vi "Change Setting.vi"(8 "error in (no error)":errorcluster, 10 "Change setting mode":T1=enum."Next", 11 "Toggle 8 in":refnum<class "Toggle 8.lvclass">) -> (0 "error out":errorcluster, 1 "Changes":cluster{"Name":string, "Value":string}[](array[cluster]), 2 "Last setting":bool, 3 "Toggle 8 out":refnum<class "Toggle 8.lvclass">)   [LabVIEW 2020, in "Toggle 8.lvclass"]
uses:
  Toggle 8.lvclass
  Controls/Change setting mode enum.ctl
  Controls/Register to Write.ctl
  PIC-device/PIC-Device.lvclass
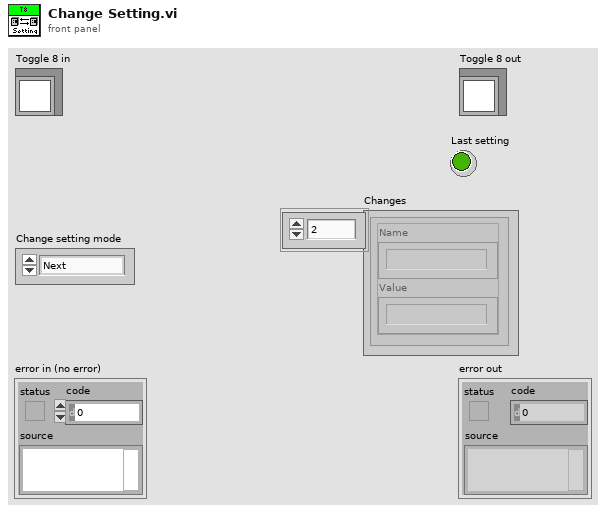
[diagram p1: front panel]
types:
  T1 = typedef "PIC-Device.lvclass/Change setting mode enum.ctl" = enum16{"Init", "Next", "Reset"}
  T2 = typedef "Toggle 8.lvclass/Test Sequence.ctl" = cluster{"CP values":string, "Charge Pump values":enum16{"CP 24V", "CP 26V", "CP 28V", "CP 30V", "CP 31V", "CP 32V", "CP 33V", "CP 34V", "CP 35V", "CP 36V", "CP 37V", "CP 38V", "CP 39V", "CP 40V", "CP 41V", "CP 42V", "CP 43V", "CP 44V", "CP 45V", "CP 46V", "CP 47V", "CP 48V", "CP 49V", "CP 50V", "CP 51V", "CP 52V", "CP 53V", "CP 54V", "CP 56V", "CP 58V", "CP 60V", "CP 62V"}[], "Charge Pump":T3[], "Control individual beams":bool, "OTP/beam values":dbl[], "Capa settings":T3[], "OTP Values string":string}
  T3 = typedef "PIC-Device.lvclass/Register to Write.ctl" = cluster{"Register":u32, "Value":u32, "Dev Address":u32, "Physical Adress":u32}
  T4 = enum16{"CP 24V", "CP 26V", "CP 28V", "CP 30V", "CP 31V", "CP 32V", "CP 33V", "CP 34V", "CP 35V", "CP 36V", "CP 37V", "CP 38V", "CP 39V", "CP 40V", "CP 41V", "CP 42V", "CP 43V", "CP 44V", "CP 45V", "CP 46V", "CP 47V", "CP 48V", "CP 49V", "CP 50V", "CP 51V", "CP 52V", "CP 53V", "CP 54V", "CP 56V", "CP 58V", "CP 60V", "CP 62V"}[]
  T5 = enum16{"CP 24V", "CP 26V", "CP 28V", "CP 30V", "CP 31V", "CP 32V", "CP 33V", "CP 34V", "CP 35V", "CP 36V", "CP 37V", "CP 38V", "CP 39V", "CP 40V", "CP 41V", "CP 42V", "CP 43V", "CP 44V", "CP 45V", "CP 46V", "CP 47V", "CP 48V", "CP 49V", "CP 50V", "CP 51V", "CP 52V", "CP 53V", "CP 54V", "CP 56V", "CP 58V", "CP 60V", "CP 62V"}
  T6 = cluster{"Register":bool, "Value":bool, "Dev Address":bool, "Physical Adress":bool}
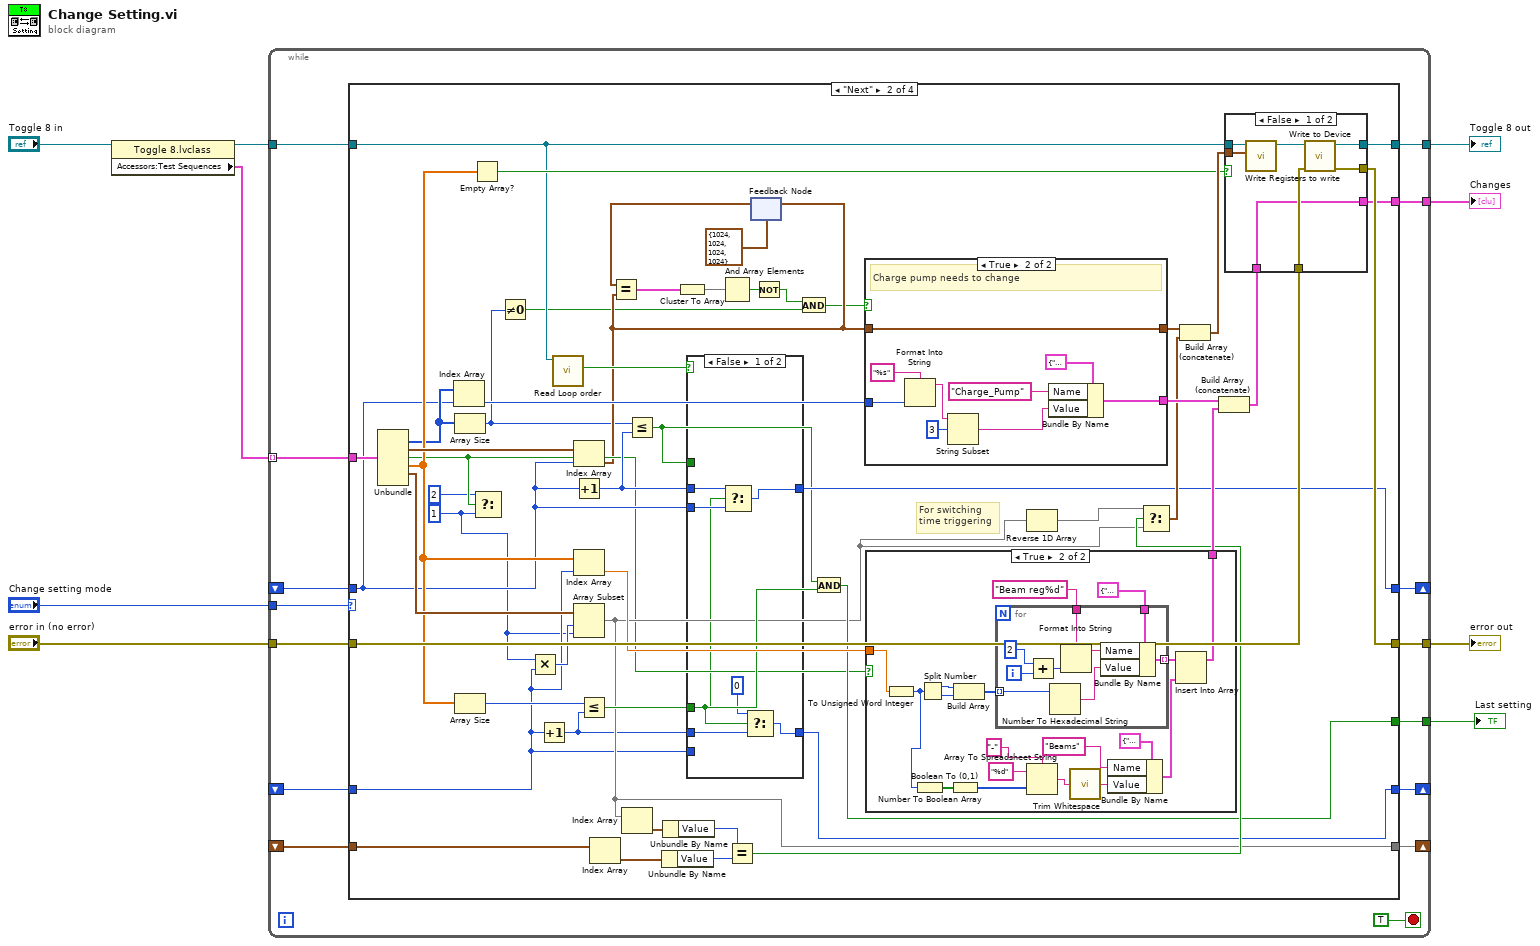
[diagram p0: block diagram]
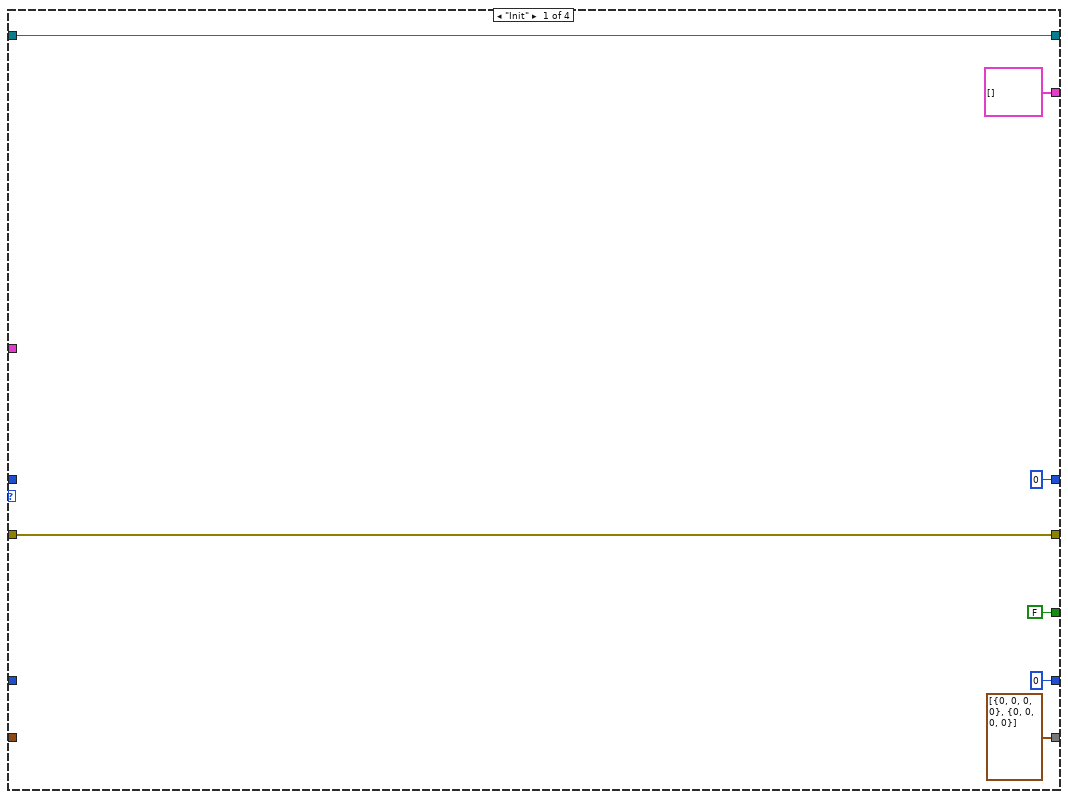
[diagram p2: hidden frame]
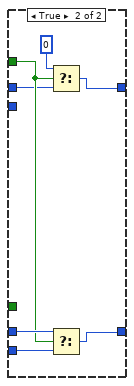
[diagram p3: hidden frame]
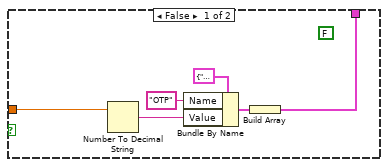
[diagram p4: hidden frame]
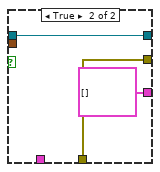
[diagram p6: hidden frame]
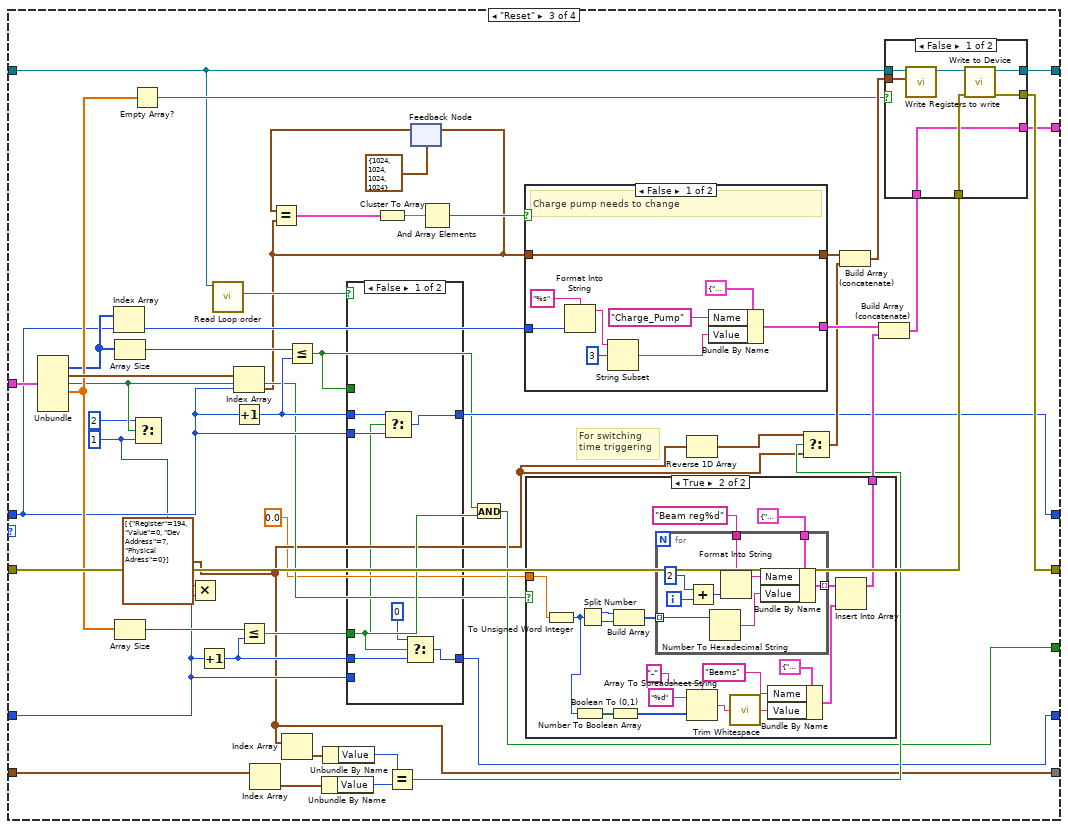
[diagram p7: hidden frame]
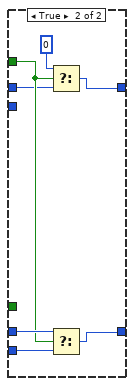
[diagram p8: hidden frame]
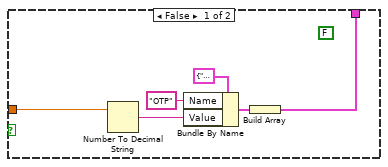
[diagram p9: hidden frame]
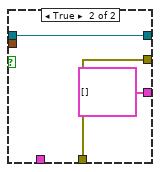
[diagram p11: hidden frame]
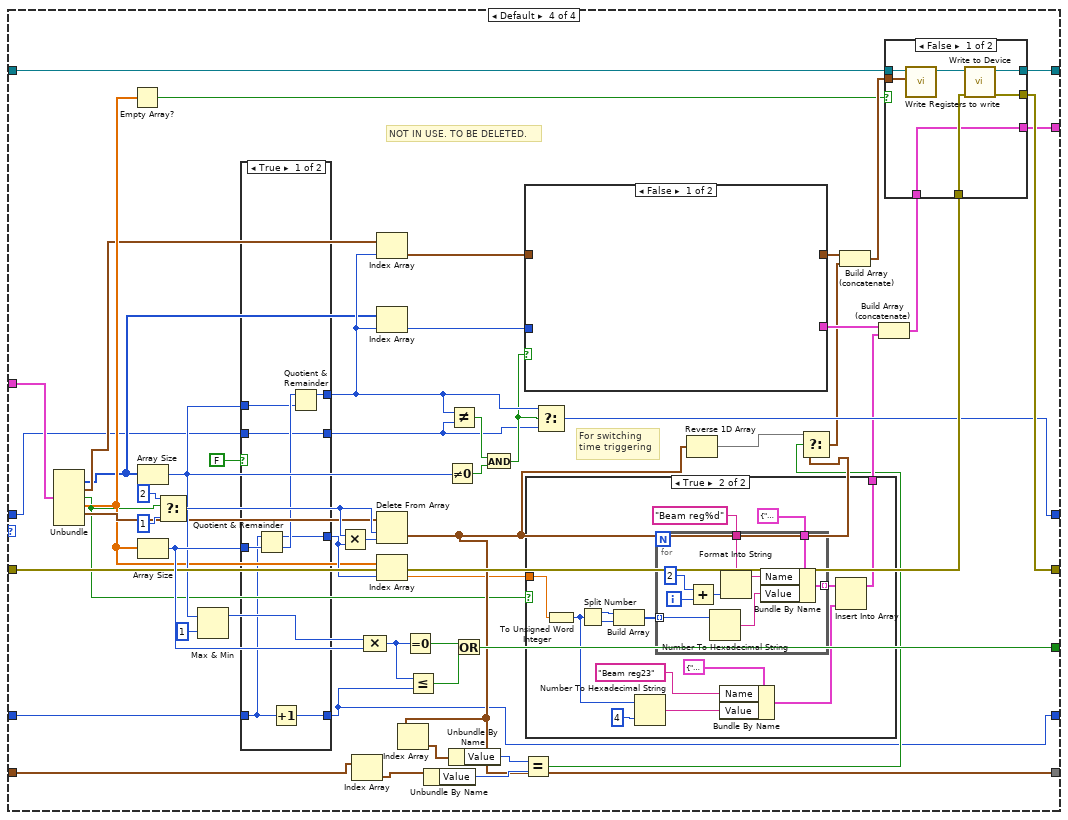
[diagram p12: hidden frame]
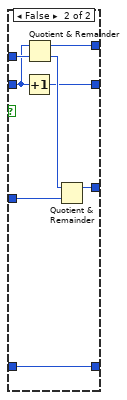
[diagram p13: hidden frame]
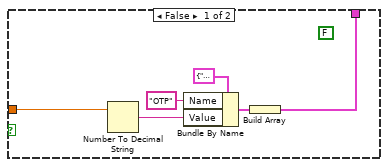
[diagram p14: hidden frame]
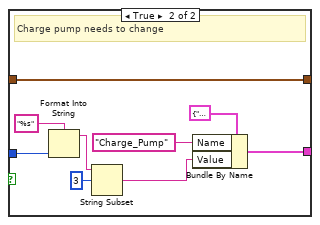
[diagram p15: hidden frame]
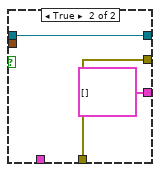
[diagram p16: hidden frame]
diagram:
  n1 = property class="Toggle 8.lvclass"(reference="Toggle 8 in") -> (reference out=w6:refnum<class "Toggle 8.lvclass">, "Accessors:Test Sequences"=w8:T2[])  [unwired: 1 in, 1 out]
  n2 = while {
    tunnel: w8 -> [w24] mode=indexing
    tunnel: "Change setting mode" -> [w22]
    shift-right: [w10] -> _
    shift-left: _ -> [w11]
    shift-right: [w21] -> _
    shift-left: _ -> [w20]
    tunnel: w6 -> [w19]
    tunnel: [w18] -> w5
    tunnel: [w17] -> w4
    tunnel: "error in (no error)" -> [w16]
    tunnel: [w15] -> w2
    tunnel: [w14] -> w1
    shift-right: [w13] -> _
    shift-left: _ -> [w12]
    stop <- TRUE stop-if-true
    n3 = case shown="\"Next\"" w22 {
      tunnel: w24 -> [_ w83 w196 w314]
      tunnel: [0 w49 w165 w264] -> w10
      tunnel: w11 -> [_ w46 w162 w265]
      tunnel: [0 w56 w170 w305] -> w21
      tunnel: w20 -> [_ w57 w171 w266]
      tunnel: w19 -> [w26 w45 w161 w311]
      tunnel: [w26 w80 w193 w310] -> w18
      tunnel: [FALSE w60 w174 w296] -> w17
      tunnel: w16 -> [w28 w79 w192 w308]
      tunnel: [w28 w78 w191 w307] -> w15
      tunnel: [cluster{"Name":string, "Value":string}[] [] w75 w188 w300] -> w14
      tunnel: [T3[] [{"Register"=0, "Value"=0, "Dev Address"=0, "Physical Adress"=0}, {"Register"=0, "Value"=0, "Dev Address"=0, "Physical Adress"=0}] ("Capa settings") w55 w151 w275] -> w13
      tunnel: w12 -> [_ w71 w184 w280]
      frame "Init" {
      }
      frame "Next" {
        w37 = 1
        # "For switching \ntime triggering"
        n4 = Unbundle(w83) -> ("Charge Pump values"=w62:T4, "Charge Pump"=w64:T3[], "Control individual beams"=w53:bool, "OTP/beam values"=w63:dbl[], "Capa settings"=w65:T3[])  [unwired: 2 out]
        n5 = Index Array(array=w62, index=w57) -> (element=w50:T5)
        n6 = Array Size(array=w62) -> (size(s)=w36:i32)
        n7 = Array Size(array=w63) -> (size(s)=w61:i32)
        n8 = Empty Array?(array=w63) -> (empty?=w81:bool)
        n9 = Select(t=2, s=w53, f=w37) -> ()  [unwired: 1 out]
        n10 = Not Equal To 0?(x=w36) -> (x != 0?=w35:bool)
        n11 = Multiply(x=w37, y=w46) -> (x*y=w51:i32)
        n12 = Increment(x=w46) -> (x+1=w48:i32)
        n13 = call-dynamic "Read Loop order.vi"("Toggle 8 in"=w45) -> ("Loop order"=w44:bool)  [unwired: 9 in, 1 out]
        n14 = Index Array(array=w64, index=w57) -> (element=w38:T3)
        n15 = Increment(x=w57) -> (x+1=w58:i32)
        n16 = Index Array(array=w63, index=w46) -> (element=w66:dbl)
        n17 = Array Subset(array=w65, index=w51, length=w37) -> (w55:T3[])
        n18 = Less Or Equal?(x=w61, y=w48) -> (x <= y?=w59:bool)
        n19 = Index Array(array=w71) -> (element=w70:T3)  [unwired: 1 in]
        n20 = Index Array(array=w55) -> (element=w54:T3)  [unwired: 1 in]
        n21 = Less Or Equal?(x=w36, y=w58) -> (x <= y?=w47:bool)
        n22 = Unbundle By Name(w70) -> ("Value"=w69:u32)
        n23 = Unbundle By Name(w54) -> ("Value"=w68:u32)
        n24 = case shown="False" w44 {
          tunnel: w59 -> [w87 _]
          tunnel: w58 -> [w90 w93]
          tunnel: w57 -> [w89 _]
          tunnel: [w84 w92] -> w56
          tunnel: [w85 w95] -> w49
          tunnel: w48 -> [w86 w97]
          tunnel: w46 -> [_ w96]
          tunnel: w47 -> [_ w94]
          frame False {
            n25 = Select(t=w90, s=w87, f=w89) -> (s? t:f=w84:i32)
            n26 = Select(t=0, s=w87, f=w86) -> (s? t:f=w85:i32)
          }
          frame True {
            n27 = Select(t=0, s=w94, f=w93) -> (s? t:f=w92:i32)
            n28 = Select(t=w97, s=w94, f=w96) -> (s? t:f=w95:i32)
          }
        }
        n29 = Equal?(x=w68, y=w69) -> (x = y?=w67:bool)
        n30 = feedback-in #1(w38) -> ()
        n31 = feedback #1(T3 {"Register"=1024, "Value"=1024, "Dev Address"=1024, "Physical Adress"=1024} ("reg cluster")) -> (w42:T3)
        n32 = Equal?(x=w42, y=w38) -> (x = y?=w41:T6)
        n33 = Cluster To Array(cluster=w41) -> (array=w40:bool[])
        n34 = And Array Elements(Boolean array=w40) -> (logical AND=w33:bool)
        n35 = Not(x=w33) -> (.not. x?=w32:bool)
        n36 = And(x=w32, y=w35) -> (x .and. y?=w34:bool)
        n37 = And(x=w47, y=w59) -> (x .and. y?=w60:bool)
        n38 = case shown="True" w34 {
          tunnel: w38 -> [_ w137]
          tunnel: w50 -> [_ w134]
          tunnel: [_ w137] -> w43
          tunnel: [_ w136] -> w77
          frame False {
          }
          frame True {
            # "Charge pump needs to change"
            n39 = Format Into String(format string="%s", w134) -> (resulting string=w133:string)  [unwired: 2 in, 1 out]
            n40 = String Subset(string=w133, offset (0)=3) -> (substring=w131:string)  [unwired: 1 in]
            n41 = Bundle By Name(cluster=cluster{"Name":string, "Value":string} {"Name"="", "Value"=""} ("Change"), "Name"="Charge_Pump", "Value"=w131) -> (w136:cluster{"Name":string, "Value":string})
          }
        }
        n42 = case shown="True" w53 {
          tunnel: [w101 w111] -> w74
          tunnel: w66 -> [w98 w117]
          frame False {
            (unwired) FALSE
            n43 = Number To Decimal String(number=w98) -> (decimal integer string=w99:string)  [unwired: 1 in]
            n44 = Bundle By Name(cluster=cluster{"Name":string, "Value":string} {"Name"="", "Value"=""} ("Change"), "Name"="OTP", "Value"=w99) -> (w102:cluster{"Name":string, "Value":string})
            n45 = Build Array(w102) -> (w101:cluster{"Name":string, "Value":string}[])
          }
          frame True {
            n46 = To Unsigned Word Integer(number=w117) -> (unsigned 16bit integer=w106:u16)
            n47 = Number To Boolean Array(number=w106) -> (Boolean array=w109:bool[])
            n48 = Split Number(x=w106) -> (hi(x)=w118:u8, lo(x)=w119:u8)
            n49 = Boolean To (0,1)(Boolean=w109) -> (0, 1=w110:i16[])
            n50 = Build Array(w118, w119) -> (w116:u8[])
            n51 = for {
              tunnel: cluster{"Name":string, "Value":string} {"Name"="", "Value"=""} ("Change") -> [w130]
              tunnel: [w129] -> w112 mode=indexing
              tunnel: "Beam reg%d" ("Name") -> [w128]
              tunnel: w116 -> [w122] mode=indexing
              i -> [w127]
              n52 = Add(x=2, y=w127) -> (x+y=w125:i32)
              n53 = Number To Hexadecimal String(2:w122) -> (0:w123:string)  [unwired: 1 in]
              n54 = Format Into String(format string=w128, w125) -> (resulting string=w124:string)  [unwired: 2 in, 1 out]
              n55 = Bundle By Name(cluster=w130, "Name"=w124, "Value"=w123) -> (w129:cluster{"Name":string, "Value":string})
            }
            n56 = Array To Spreadsheet String(delimiter (Tab)="-", array=w110, 3:"%d" ("format string")) -> (spreadsheet string=w105:string)
            n57 = call <vilib>:"Trim Whitespace.vi"("string"=w105) -> ("trimmed string"=w104:string)  [unwired: 1 in]
            n58 = Bundle By Name(cluster=cluster{"Name":string, "Value":string} {"Name"="", "Value"=""} ("Change"), "Name"="Beams", "Value"=w104) -> (w113:cluster{"Name":string, "Value":string})
            n59 = Insert Into Array(array=w112, new element=w113) -> (w111:cluster{"Name":string, "Value":string}[])  [unwired: 1 in]
          }
        }
        n60 = Reverse 1D Array(array=w55) -> (reversed array=w73:T3[])
        n61 = Select(t=w73, s=w67, f=w55) -> (s? t:f=w72:T3[])
        n62 = Build Array (concatenate)(w43, w72) -> (w82:T3[])
        n63 = Build Array (concatenate)(w77, w74) -> (w76:cluster{"Name":string, "Value":string}[])
        n64 = case shown="False" w81 {
          tunnel: w45 -> [w146 w149]
          tunnel: w82 -> [w145 _]
          tunnel: [w143 w149] -> w80
          tunnel: [w142 w147] -> w78
          tunnel: [w140 cluster{"Name":string, "Value":string}[] []] -> w75
          tunnel: w79 -> [w141 w147]
          tunnel: w76 -> [w140 _]
          frame False {
            n65 = call-dynamic "Write Registers to write.vi"("Registers to write"=w145, "Device in"=w146) -> ("Device out"=w144:refnum<class "Toggle 8.lvclass">)  [unwired: 9 in]
            n66 = call-dynamic "Write to Device.vi"("error in (no error)"=w141, "Device in"=w144) -> ("error out"=w142:errorcluster, "Device out"=w143:refnum<class "Toggle 8.lvclass">)  [unwired: 7 in, 1 out]
          }
          frame True {
          }
        }
      }
      frame "Reset" {
        w151 = T3[] [{"Register"=194, "Value"=0, "Dev Address"=7, "Physical Adress"=0}] ("Capa settings")
        w152 = 1
        # "For switching \ntime triggering"
        n67 = Unbundle(w196) -> ("Charge Pump values"=w177:T4, "Charge Pump"=w179:T3[], "Control individual beams"=w168:bool, "OTP/beam values"=w178:dbl[])  [unwired: 3 out]
        n68 = Index Array(array=w177, index=w171) -> (element=w166:T5)
        n69 = Array Size(array=w177) -> (size(s)=w175:i32)
        n70 = Array Size(array=w178) -> (size(s)=w176:i32)
        n71 = Empty Array?(array=w178) -> (empty?=w194:bool)
        n72 = Select(t=2, s=w168, f=w152) -> ()  [unwired: 1 out]
        n73 = Multiply(x=w152, y=w162) -> ()  [unwired: 1 out]
        n74 = Increment(x=w162) -> (x+1=w164:i32)
        n75 = call-dynamic "Read Loop order.vi"("Toggle 8 in"=w161) -> ("Loop order"=w160:bool)  [unwired: 9 in, 1 out]
        n76 = Index Array(array=w179, index=w171) -> (element=w153:T3)
        n77 = Increment(x=w171) -> (x+1=w172:i32)
        n78 = Less Or Equal?(x=w176, y=w164) -> (x <= y?=w173:bool)
        n79 = Index Array(array=w184) -> (element=w183:T3)  [unwired: 1 in]
        n80 = Index Array(array=w151) -> (element=w169:T3)  [unwired: 1 in]
        n81 = Less Or Equal?(x=w175, y=w172) -> (x <= y?=w163:bool)
        n82 = Unbundle By Name(w183) -> ("Value"=w182:u32)
        n83 = Unbundle By Name(w169) -> ("Value"=w181:u32)
        n84 = case shown="False" w160 {
          tunnel: w173 -> [w200 _]
          tunnel: w172 -> [w203 w206]
          tunnel: w171 -> [w202 _]
          tunnel: [w197 w205] -> w170
          tunnel: [w198 w208] -> w165
          tunnel: w164 -> [w199 w210]
          tunnel: w162 -> [_ w209]
          tunnel: w163 -> [_ w207]
          frame False {
            n85 = Select(t=w203, s=w200, f=w202) -> (s? t:f=w197:i32)
            n86 = Select(t=0, s=w200, f=w199) -> (s? t:f=w198:i32)
          }
          frame True {
            n87 = Select(t=0, s=w207, f=w206) -> (s? t:f=w205:i32)
            n88 = Select(t=w210, s=w207, f=w209) -> (s? t:f=w208:i32)
          }
        }
        n89 = Equal?(x=w181, y=w182) -> (x = y?=w180:bool)
        n90 = feedback-in #2(w153) -> ()
        n91 = feedback #2(T3 {"Register"=1024, "Value"=1024, "Dev Address"=1024, "Physical Adress"=1024} ("reg cluster")) -> (w158:T3)
        n92 = Equal?(x=w158, y=w153) -> (x = y?=w157:T6)
        n93 = Cluster To Array(cluster=w157) -> (array=w156:bool[])
        n94 = And Array Elements(Boolean array=w156) -> (logical AND=w155:bool)
        n95 = And(x=w163, y=w173) -> (x .and. y?=w174:bool)
        n96 = case shown="False" w155 {
          tunnel: w153 -> [w250 _]
          tunnel: w166 -> [w247 _]
          tunnel: [w250 _] -> w159
          tunnel: [w249 _] -> w190
          frame False {
            # "Charge pump needs to change"
            n97 = Format Into String(format string="%s", w247) -> (resulting string=w246:string)  [unwired: 2 in, 1 out]
            n98 = String Subset(string=w246, offset (0)=3) -> (substring=w244:string)  [unwired: 1 in]
            n99 = Bundle By Name(cluster=cluster{"Name":string, "Value":string} {"Name"="", "Value"=""} ("Change"), "Name"="Charge_Pump", "Value"=w244) -> (w249:cluster{"Name":string, "Value":string})
          }
          frame True {
          }
        }
        n100 = case shown="True" w168 {
          tunnel: [w214 w224] -> w187
          tunnel: 0.0 ("OTP/beam value") -> [w211 w230]
          frame False {
            (unwired) FALSE
            n101 = Number To Decimal String(number=w211) -> (decimal integer string=w212:string)  [unwired: 1 in]
            n102 = Bundle By Name(cluster=cluster{"Name":string, "Value":string} {"Name"="", "Value"=""} ("Change"), "Name"="OTP", "Value"=w212) -> (w215:cluster{"Name":string, "Value":string})
            n103 = Build Array(w215) -> (w214:cluster{"Name":string, "Value":string}[])
          }
          frame True {
            n104 = To Unsigned Word Integer(number=w230) -> (unsigned 16bit integer=w219:u16)
            n105 = Number To Boolean Array(number=w219) -> (Boolean array=w222:bool[])
            n106 = Split Number(x=w219) -> (hi(x)=w231:u8, lo(x)=w232:u8)
            n107 = Boolean To (0,1)(Boolean=w222) -> (0, 1=w223:i16[])
            n108 = Build Array(w231, w232) -> (w229:u8[])
            n109 = for {
              tunnel: cluster{"Name":string, "Value":string} {"Name"="", "Value"=""} ("Change") -> [w243]
              tunnel: [w242] -> w225 mode=indexing
              tunnel: "Beam reg%d" ("Name") -> [w241]
              tunnel: w229 -> [w235] mode=indexing
              i -> [w240]
              n110 = Add(x=2, y=w240) -> (x+y=w238:i32)
              n111 = Number To Hexadecimal String(2:w235) -> (0:w236:string)  [unwired: 1 in]
              n112 = Format Into String(format string=w241, w238) -> (resulting string=w237:string)  [unwired: 2 in, 1 out]
              n113 = Bundle By Name(cluster=w243, "Name"=w237, "Value"=w236) -> (w242:cluster{"Name":string, "Value":string})
            }
            n114 = Array To Spreadsheet String(delimiter (Tab)="-", array=w223, 3:"%d" ("format string")) -> (spreadsheet string=w218:string)
            n115 = call <vilib>:"Trim Whitespace.vi"("string"=w218) -> ("trimmed string"=w217:string)  [unwired: 1 in]
            n116 = Bundle By Name(cluster=cluster{"Name":string, "Value":string} {"Name"="", "Value"=""} ("Change"), "Name"="Beams", "Value"=w217) -> (w226:cluster{"Name":string, "Value":string})
            n117 = Insert Into Array(array=w225, new element=w226) -> (w224:cluster{"Name":string, "Value":string}[])  [unwired: 1 in]
          }
        }
        n118 = Reverse 1D Array(array=w151) -> (reversed array=w186:T3[])
        n119 = Select(t=w186, s=w180, f=w151) -> (s? t:f=w185:T3[])
        n120 = Build Array (concatenate)(w159, w185) -> (w195:T3[])
        n121 = Build Array (concatenate)(w190, w187) -> (w189:cluster{"Name":string, "Value":string}[])
        n122 = case shown="False" w194 {
          tunnel: w161 -> [w259 w262]
          tunnel: w195 -> [w258 _]
          tunnel: [w256 w262] -> w193
          tunnel: [w255 w260] -> w191
          tunnel: [w253 cluster{"Name":string, "Value":string}[] []] -> w188
          tunnel: w192 -> [w254 w260]
          tunnel: w189 -> [w253 _]
          frame False {
            n123 = call-dynamic "Write Registers to write.vi"("Registers to write"=w258, "Device in"=w259) -> ("Device out"=w257:refnum<class "Toggle 8.lvclass">)  [unwired: 9 in]
            n124 = call-dynamic "Write to Device.vi"("error in (no error)"=w254, "Device in"=w257) -> ("error out"=w255:errorcluster, "Device out"=w256:refnum<class "Toggle 8.lvclass">)  [unwired: 7 in, 1 out]
          }
          frame True {
          }
        }
      }
      frame Default {
        # "NOT IN USE. TO BE DELETED."
        # "For switching \ntime triggering"
        n125 = Unbundle(w314) -> ("Charge Pump values"=w268:T4, "Charge Pump"=w269:T3[], "Control individual beams"=w270:bool, "OTP/beam values"=w271:dbl[], "Capa settings"=w272:T3[])  [unwired: 2 out]
        n126 = Empty Array?(array=w271) -> (empty?=w312:bool)
        n127 = Array Size(array=w268) -> (size(s)=w287:i32)
        n128 = Array Size(array=w271) -> (size(s)=w309:i32)
        n129 = Select(t=2, s=w270, f=1) -> (s? t:f=w293:i32)
        n130 = Max & Min(x=w287, y=1) -> (max(x,y)=w289:i32)  [unwired: 1 out]
        n131 = case shown="True" FALSE {
          tunnel: w309 -> [w321 w330]
          tunnel: [w320 w329] -> w292
          tunnel: [w319 w328] -> w290
          tunnel: w287 -> [w318 w327]
          tunnel: w266 -> [w316 w324]
          tunnel: w265 -> [w315 w325]
          tunnel: [w317 w325] -> w264
          tunnel: [w316 w323] -> w263
          frame True {
            n132 = Quotient & Remainder(x=w315, y=w321) -> (x-y*floor(x/y)=w320:i32, floor(x/y)=w322:i32)
            n133 = Increment(x=w315) -> (x+1=w317:i32)
            n134 = Quotient & Remainder(x=w322, y=w318) -> (x-y*floor(x/y)=w319:i32)  [unwired: 1 out]
          }
          frame False {
            n135 = Increment(x=w324) -> (x+1=w323:i32)
            n136 = Quotient & Remainder(x=w324, y=w327) -> (x-y*floor(x/y)=w328:i32, floor(x/y)=w326:i32)
            n137 = Quotient & Remainder(x=w326, y=w330) -> (x-y*floor(x/y)=w329:i32)  [unwired: 1 out]
          }
        }
        n138 = Multiply(x=w293, y=w292) -> (x*y=w291:i32)
        n139 = Index Array(array=w280) -> (element=w279:T3)  [unwired: 1 in]
        n140 = Compound Arithmetic op=MULTIPLY(w289, w309) -> (w299:i32)
        n141 = Index Array(array=w269, index=w290) -> (element=w304:T3)
        n142 = Index Array(array=w268, index=w290) -> (element=w306:T5)
        n143 = Delete From Array(array=w272, length=w293, index=w291) -> (deleted portion=w275:T3[])  [unwired: 1 out]
        n144 = Index Array(array=w271, index=w292) -> (element=w273:dbl)
        n145 = Index Array(array=w275) -> (element=w276:T3)  [unwired: 1 in]
        n146 = Equal To 0?(x=w299) -> (x = 0?=w298:bool)
        n147 = Less Or Equal?(x=w299, y=w264) -> (x <= y?=w297:bool)
        n148 = Unbundle By Name(w279) -> ("Value"=w278:u32)
        n149 = Not Equal To 0?(x=w287) -> (x != 0?=w286:bool)
        n150 = Not Equal?(x=w290, y=w263) -> (x != y?=w285:bool)
        n151 = Unbundle By Name(w276) -> ("Value"=w277:u32)
        n152 = Or(x=w298, y=w297) -> (x .or. y?=w296:bool)
        n153 = And(x=w285, y=w286) -> (x .and. y?=w284:bool)
        n154 = Equal?(x=w277, y=w278) -> (x = y?=w274:bool)
        n155 = case shown="False" w284 {
          tunnel: w304 -> [_ w366]
          tunnel: w306 -> [_ w363]
          tunnel: [_ w366] -> w303
          tunnel: [_ w365] -> w302
          frame False {
          }
          frame True {
            # "Charge pump needs to change"
            n156 = Format Into String(format string="%s", w363) -> (resulting string=w362:string)  [unwired: 2 in, 1 out]
            n157 = String Subset(string=w362, offset (0)=3) -> (substring=w360:string)  [unwired: 1 in]
            n158 = Bundle By Name(cluster=cluster{"Name":string, "Value":string} {"Name"="", "Value"=""} ("Change"), "Name"="Charge_Pump", "Value"=w360) -> (w365:cluster{"Name":string, "Value":string})
          }
        }
        n159 = case shown="True" w270 {
          tunnel: [w334 w338] -> w283
          tunnel: w273 -> [w331 w346]
          frame False {
            (unwired) FALSE
            n160 = Number To Decimal String(number=w331) -> (decimal integer string=w332:string)  [unwired: 1 in]
            n161 = Bundle By Name(cluster=cluster{"Name":string, "Value":string} {"Name"="", "Value"=""} ("Change"), "Name"="OTP", "Value"=w332) -> (w335:cluster{"Name":string, "Value":string})
            n162 = Build Array(w335) -> (w334:cluster{"Name":string, "Value":string}[])
          }
          frame True {
            n163 = To Unsigned Word Integer(number=w346) -> (unsigned 16bit integer=w337:u16)
            n164 = Split Number(x=w337) -> (hi(x)=w347:u8, lo(x)=w348:u8)
            n165 = Build Array(w347, w348) -> (w345:u8[])
            n166 = Number To Hexadecimal String(1:i16 4 ("width (-)"), 2:w337) -> (0:w343:string)
            n167 = for {
              tunnel: cluster{"Name":string, "Value":string} {"Name"="", "Value"=""} ("Change") -> [w359]
              tunnel: [w358] -> w339 mode=indexing
              tunnel: "Beam reg%d" ("Name") -> [w357]
              tunnel: w345 -> [w351] mode=indexing
              i -> [w356]
              n168 = Add(x=2, y=w356) -> (x+y=w354:i32)
              n169 = Number To Hexadecimal String(2:w351) -> (0:w352:string)  [unwired: 1 in]
              n170 = Format Into String(format string=w357, w354) -> (resulting string=w353:string)  [unwired: 2 in, 1 out]
              n171 = Bundle By Name(cluster=w359, "Name"=w353, "Value"=w352) -> (w358:cluster{"Name":string, "Value":string})
            }
            n172 = Bundle By Name(cluster=cluster{"Name":string, "Value":string} {"Name"="", "Value"=""} ("Change"), "Name"="Beam reg23", "Value"=w343) -> (w341:cluster{"Name":string, "Value":string})
            n173 = Insert Into Array(array=w339, new element=w341) -> (w338:cluster{"Name":string, "Value":string}[])  [unwired: 1 in]
          }
        }
        n174 = Select(t=w290, s=w284, f=w263) -> (s? t:f=w305:i32)
        n175 = Reverse 1D Array(array=w275) -> (reversed array=w282:T3[])
        n176 = Select(t=w282, s=w274, f=w275) -> (s? t:f=w281:T3[])
        n177 = Build Array (concatenate)(w303, w281) -> (w313:T3[])
        n178 = Build Array (concatenate)(w302, w283) -> (w301:cluster{"Name":string, "Value":string}[])
        n179 = case shown="False" w312 {
          tunnel: w311 -> [w375 w378]
          tunnel: w313 -> [w374 _]
          tunnel: [w372 w378] -> w310
          tunnel: [w371 w376] -> w307
          tunnel: [w369 cluster{"Name":string, "Value":string}[] []] -> w300
          tunnel: w308 -> [w370 w376]
          tunnel: w301 -> [w369 _]
          frame False {
            n180 = call-dynamic "Write Registers to write.vi"("Registers to write"=w374, "Device in"=w375) -> ("Device out"=w373:refnum<class "Toggle 8.lvclass">)  [unwired: 9 in]
            n181 = call-dynamic "Write to Device.vi"("error in (no error)"=w370, "Device in"=w373) -> ("error out"=w371:errorcluster, "Device out"=w372:refnum<class "Toggle 8.lvclass">)  [unwired: 7 in, 1 out]
          }
          frame True {
          }
        }
      }
    }
  }
  "error out" <- w2
  "Toggle 8 out" <- w5
  "Changes" <- w1
  "Last setting" <- w4
